vi "A1_Stop_VariableLocal.vi"() -> ()   [LabVIEW 2025]
panel:
  in  "stop":bool
  out "Boolean 4":bool
  out "Boolean":bool
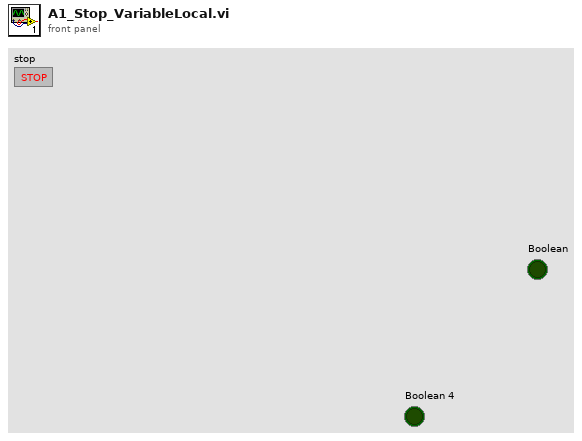
[diagram p1: front panel]
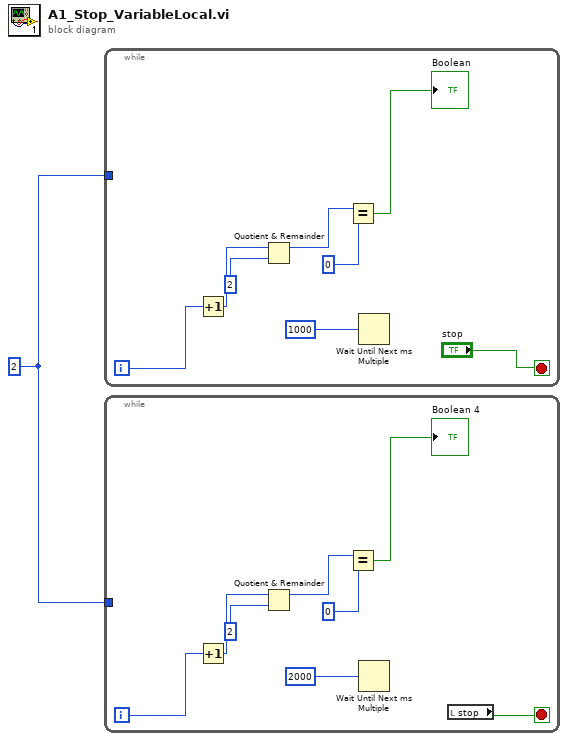
[diagram p0: block diagram]
diagram:
  w1 = 2
  n1 = while {
    tunnel: w1 -> [_]
    i -> [w9]
    stop <- "stop" stop-if-true
    n2 = Increment(x=w9) -> (x+1=w8:i32)
    n3 = Quotient & Remainder(x=w8, y=2) -> (x-y*floor(x/y)=w6:i32)  [unwired: 1 out]
    n4 = Equal?(x=w6, y=0) -> (x = y?=→"Boolean":bool)
    n5 = Wait Until Next ms Multiple(millisecond multiple=u32 1000) -> ()  [unwired: 1 out]
  }
  n6 = while {
    tunnel: [w10] -> _
    tunnel: w1 -> [w10]
    i -> [w18]
    stop <- w11 stop-if-true
    n7 = Increment(x=w18) -> (x+1=w17:i32)
    n8 = Quotient & Remainder(x=w17, y=2) -> (x-y*floor(x/y)=w15:i32)  [unwired: 1 out]
    n9 = Equal?(x=w15, y=0) -> (x = y?=→"Boolean 4":bool)
    n10 = Wait Until Next ms Multiple(millisecond multiple=u32 2000) -> ()  [unwired: 1 out]
    n11 = local read "stop"() -> (w11:bool)
  }
